vi "decision_path.vi"(8 "error in (no error)":errorcluster, 11 "Interface_decision_path in":refnum<class "Interface_decision_path.lvclass">) -> (0 "error out":errorcluster, 2 "out":T1, 3 "Interface_decision_path out":refnum<class "Interface_decision_path.lvclass">)   [LabVIEW 2020, in "Interface_decision_path.lvclass"]
doc: "Return the decision path."
uses:
  Interface_decision_path.lvclass
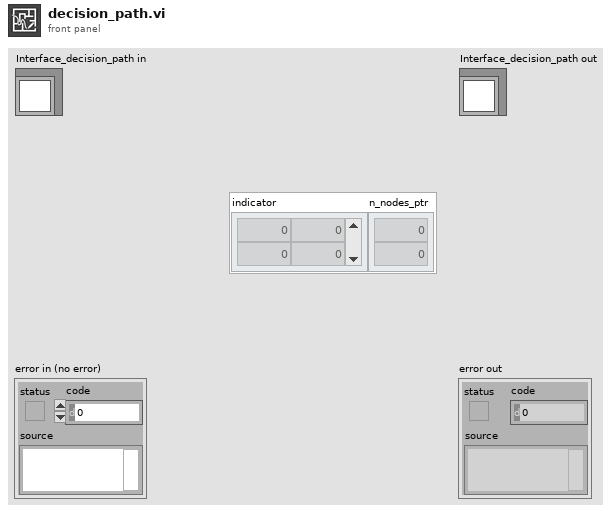
[diagram p1: front panel]
types:
  T1 = cluster{"indicator":dbl[][], "n_nodes_ptr":dbl[]}
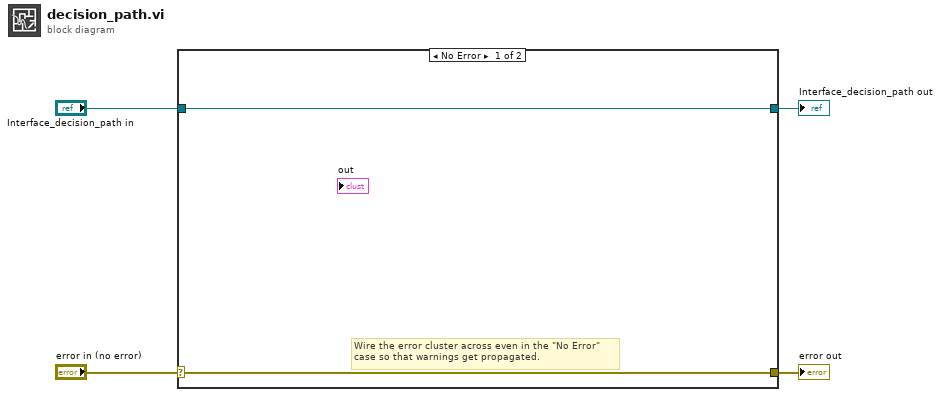
[diagram p0: block diagram]
diagram:
  n1 = case shown="No Error" "error in (no error)" {
    selector: "error in (no error)" -> [w5 w8]
    tunnel: [w5 w8] -> w3
    tunnel: [w6 w7] -> w1
    tunnel: "Interface_decision_path in" -> [w6 w7]
    frame No Error {
      # "Wire the error cluster across even in the \"No Error\"\ncase so that warnings get propagated."
    }
    frame Error {
    }
  }
  "error out" <- w3
  "Interface_decision_path out" <- w1
